vi "RelativePositionCombined_KCubeDCServo.vi"(4 "stepSize":dbl, 6 "Backward Button":bool, 7 "lower limit":dbl, 9 "Forward Button":bool, 10 "upper limit":dbl, 11 ".NET Refnum in":refnum<k24>) -> (1 "backward step size":dbl, 2 "backward position response limit":string, 3 "forward step size":dbl, 5 "forward position response limit":string)   [LabVIEW 2019]
doc: "set, get, and run relative position values for dc servo motor. also can set stage limits"
uses:
  D:/Victor Sun/optical trap control/Kinesis/ThorLabs.MotionControl.KCube.DCServoCLI.dll
  Kinesis/ThorLabs.MotionControl.KCube.DCServoCLI.dll
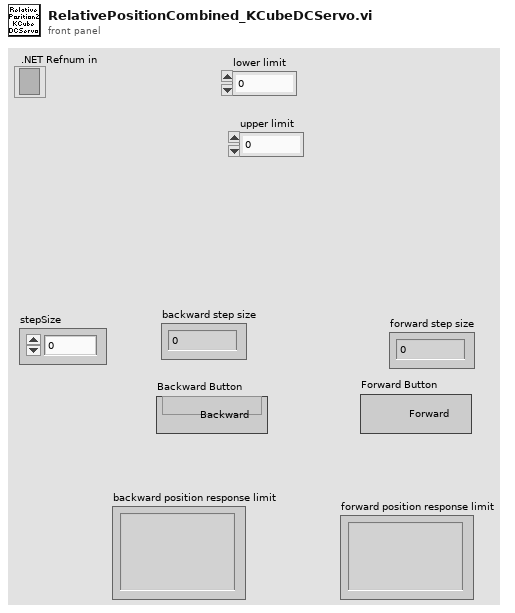
[diagram p1: front panel]
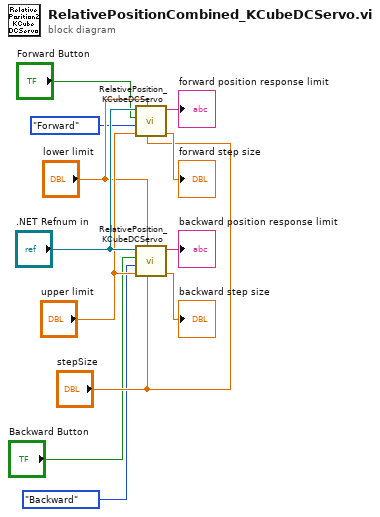
[diagram p0: block diagram]
diagram:
  n1 = call "RelativePosition_KCubeDCServo.vi"("set jog step size"="stepSize", "lower limit"="lower limit", "upper limit"="upper limit", "Direction Control"=enum16{"Backward", "Forward"}."Forward" ("Enum"), "direction button"="Forward Button", ".NET Refnum in"=".NET Refnum in") -> ("GetJogStepSize"=→"forward step size":dbl, "error output"=→"forward position response limit":string)  [unwired: 4 in]
  n2 = call "RelativePosition_KCubeDCServo.vi"("set jog step size"="stepSize", "lower limit"="lower limit", "upper limit"="upper limit", "Direction Control"=enum16{"Backward", "Forward"}."Backward", "direction button"="Backward Button", ".NET Refnum in"=".NET Refnum in") -> ("GetJogStepSize"=→"backward step size":dbl, "error output"=→"backward position response limit":string)  [unwired: 4 in]
